vi "New Parameter Message.vi"(8 "error in (no error)":errorcluster, 10 "New parameter":variant, 11 "Temperature Controller in":refnum<class "Temperature Controller.lvclass">) -> (0 "error out":errorcluster, 2 "New Parameter Message":T1, 3 "Temperature Controller out":refnum<class "Temperature Controller.lvclass">)   [LabVIEW 2020, in "RxnRover.lvlib" / "Temperature Controller.lvclass"]
doc: "Dynamic dispatch for each child controller type to provide it's proper message for setting a new parameter value (setpoint)."
uses:
  Temperature Controller.lvclass
  <userlib>/RxnRover/DynamicReentrant/src/Type Defs/Message.ctl
  <userlib>/RxnRover/DynamicReentrant/Dynamic Reentrant.lvlib
  RxnRover.lvlib
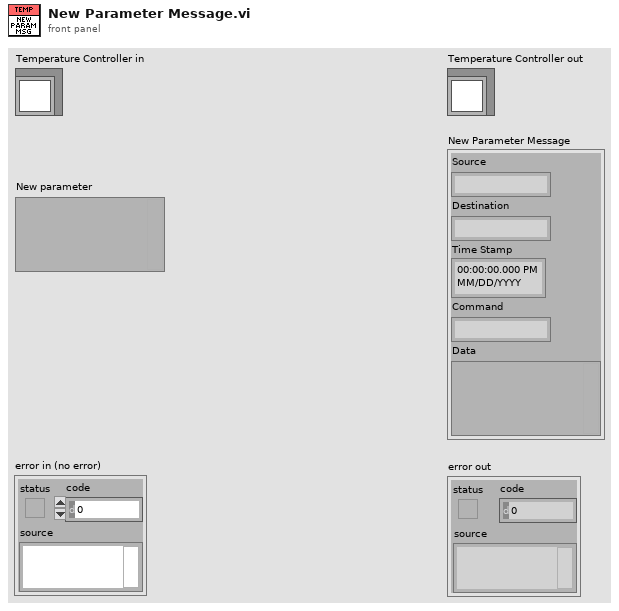
[diagram p1: front panel]
types:
  T1 = typedef "Dynamic Reentrant.lvlib/Message.ctl" = cluster{"Source":string, "Destination":string, "Time Stamp":timestamp, "Command":string, "Data":variant}
  T2 = typedef "RxnRover.lvlib/Supported Parameter Variant Types.ctl" = enum16{"Unsupported", "Numeric", "Boolean", "String", "Path"}
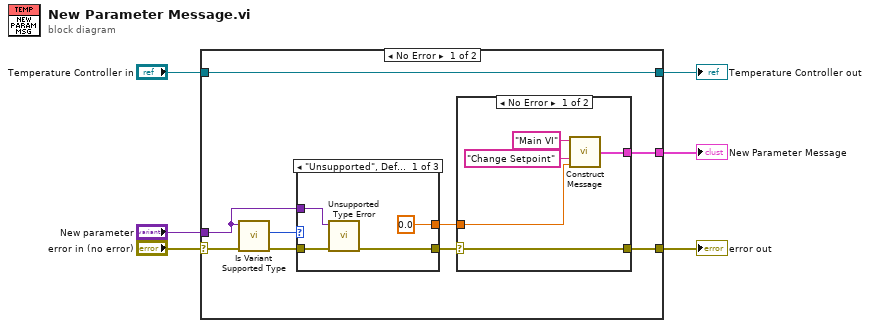
[diagram p0: block diagram]
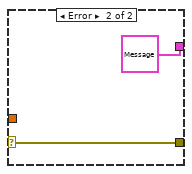
[diagram p2: hidden frame]
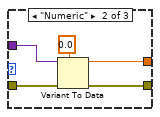
[diagram p3: hidden frame]
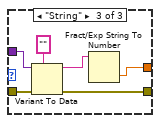
[diagram p4: hidden frame]
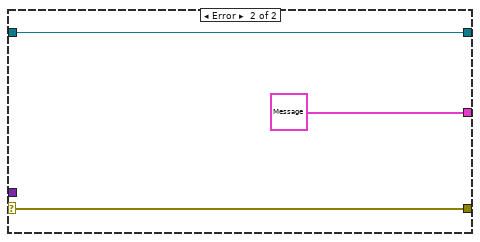
[diagram p5: hidden frame]
diagram:
  n1 = case shown="No Error" "error in (no error)" {
    selector: "error in (no error)" -> [w11 w39]
    tunnel: "New parameter" -> [w10 _]
    tunnel: [w15 T1 {"Source"="", "Destination"="", "Time Stamp"=timestamp(0 s since 1904-01-01), "Command"="", "Data"=variant} ("output cluster")] -> w5
    tunnel: [w8 w39] -> w4
    tunnel: "Temperature Controller in" -> [w14 w38]
    tunnel: [w14 w38] -> w1
    frame No Error {
      n2 = call "Is Variant Supported Type.vi"("error in (no error)"=w11, "variant"=w10) -> ("error out"=w13:errorcluster, "Type"=w12:T2)  [unwired: 7 in, 1 out]
      n3 = case shown="\"Unsupported\", Default" w12 {
        tunnel: w10 -> [w24 w31 w34]
        tunnel: [0.0 w29 w33] -> w7
        tunnel: [w25 w28 w36] -> w9
        tunnel: w13 -> [w23 w27 w37]
        frame "Unsupported", Default {
          n4 = call "Unsupported Type Error.vi"("error in (no error)"=w23, "Variant"=w24) -> ("Unsupported Parameter Variant Type"=w25:errorcluster)  [unwired: 9 in]
        }
        frame "Numeric" {
          n5 = Variant To Data(error in=w27, type=0.0, Variant=w31) -> (data=w29:dbl, error out=w28:errorcluster)
        }
        frame "String" {
          n6 = Variant To Data(error in=w37, type="", Variant=w34) -> (data=w32:string, error out=w36:errorcluster)
          n7 = Fract/Exp String To Number(string=w32) -> (number=w33:dbl)  [unwired: 3 in, 1 out]
        }
      }
      n8 = case shown="No Error" w9 {
        selector: w9 -> [w17 w21]
        tunnel: [w20 T1 {"Source"="", "Destination"="", "Time Stamp"=timestamp(0 s since 1904-01-01), "Command"="", "Data"=variant} ("Message Cluster")] -> w15
        tunnel: [w17 w21] -> w8
        tunnel: w7 -> [w16 _]
        frame No Error {
          n9 = call <userlib>:"Construct Message.vi"("Data"=w16, "Command"="Change Setpoint", "Source"="Main VI") -> ("Message Cluster"=w20:T1)  [unwired: 3 in]
        }
        frame Error {
        }
      }
    }
    frame Error {
    }
  }
  "error out" <- w4
  "Temperature Controller out" <- w1
  "New Parameter Message" <- w5
